vi "ON-OFF cooler.vi"(8 "error in (no error)":errorcluster, 10 "ON/OFF":bool, 11 "UV-VIS in":refnum<class "UV-VIS.lvclass">) -> (0 "error out":errorcluster, 3 "UV-VIS out":refnum<class "UV-VIS.lvclass">)   [LabVIEW 2015, in "UV-VIS.lvclass"]
uses:
  UV-VIS.lvclass
  Detector.lvclass/Detector.ctl
  Detector.lvclass
panel:
  out "DLL error code":u32
  out "DLL error code":u32
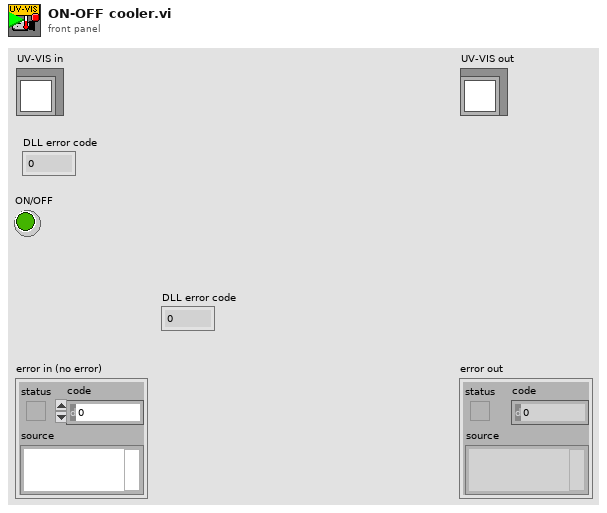
[diagram p1: front panel]
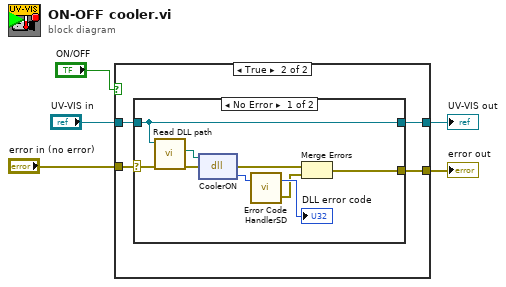
[diagram p0: block diagram]
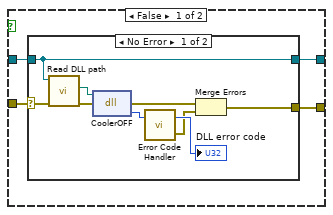
[diagram p2: hidden frame]
diagram:
  n1 = case shown="True" "ON/OFF" {
    tunnel: "error in (no error)" -> [w6 w24]
    tunnel: "UV-VIS in" -> [w7 w23]
    tunnel: [w8 w22] -> w3
    tunnel: [w9 w21] -> w2
    frame False {
      n2 = case shown="No Error" w6 {
        selector: w6 -> [w15 w20]
        tunnel: [w12 w20] -> w9
        tunnel: [w16 w19] -> w8
        tunnel: w7 -> [w16 w19]
        frame No Error {
          n3 = call "Read DLL path.vi"("error in (no error)"=w15, "Detector in"=w16) -> ("error out"=w14:errorcluster, "DLL path"=w11:path)  [unwired: 7 in, 1 out]
          n4 = dll-call lib="S:/TRANCON/DLL/Atmcd32d.dll" fn="CoolerOFF"(path in=w11, error in=w14) -> (error out=w13:errorcluster, "return type"=w18:u32)  [unwired: 1 in, 1 out]
          n5 = call "Error Code Handler.vi"("DLL error code"=w18) -> ("error out"=w10:errorcluster, "dup DLL error code"=→"DLL error code":u32)  [unwired: 1 in]
          n6 = Merge Errors(w13, w10) -> (w12:errorcluster)
        }
        frame Error {
        }
      }
    }
    frame True {
      n7 = case shown="No Error" w24 {
        selector: w24 -> [w30 w35]
        tunnel: [w25 w35] -> w21
        tunnel: [w29 w34] -> w22
        tunnel: w23 -> [w29 w34]
        frame No Error {
          n8 = call "Read DLL path.vi"("error in (no error)"=w30, "Detector in"=w29) -> ("error out"=w27:errorcluster, "DLL path"=w28:path)  [unwired: 7 in, 1 out]
          n9 = dll-call lib="S:/TRANCON/DLL/Atmcd32d.dll" fn="CoolerON"(path in=w28, error in=w27) -> (error out=w31:errorcluster, "return type"=w33:u32)  [unwired: 1 in, 1 out]
          n10 = call "Error Code HandlerSD.vi"("DLL error code"=w33) -> ("error out"=w26:errorcluster, "dup DLL error code"=→"DLL error code":u32)  [unwired: 1 in]
          n11 = Merge Errors(w31, w26) -> (w25:errorcluster)
        }
        frame Error {
        }
      }
    }
  }
  "error out" <- w2
  "UV-VIS out" <- w3
